vi "GeneralDataRequest new.vi"(6 "Enable":bool, 7 "Ring":u16(ring) items=["PID filter"=3, "Normalized"=2, "Averaged"=1, "RAW"=0], 8 "error in (no error)":errorcluster, 10 "Cluster":T1, 11 "VISA Refnum in":refnum<visa-resource-name>) -> (0 "error out":errorcluster, 3 "Holding Registers":dbl[](array[numeric]))   [LabVIEW 2020]
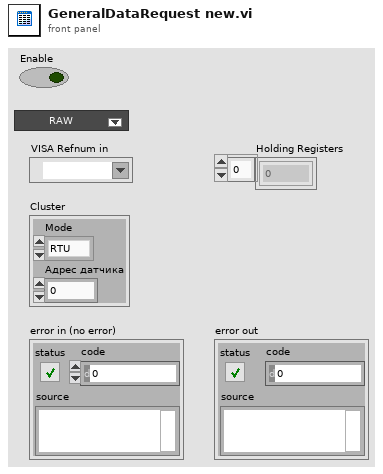
[diagram p1: front panel]
types:
  T1 = cluster{"Mode":enum16{"RTU", "ASCII"}, "Адрес датчика":u16}
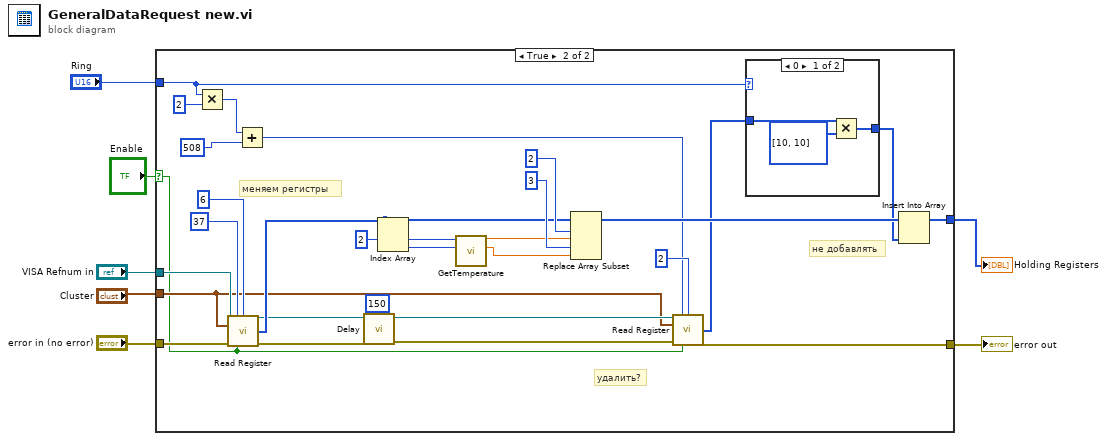
[diagram p0: block diagram]
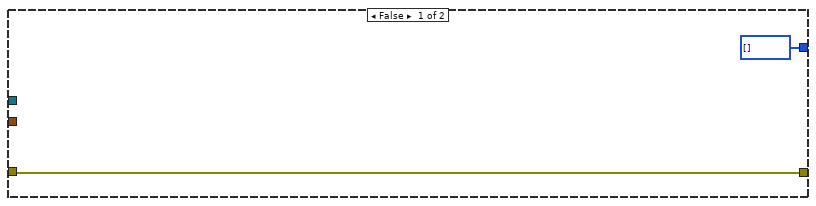
[diagram p2: hidden frame]
diagram:
  n1 = case shown="True" "Enable" {
    selector: "Enable" -> [_ w10]
    tunnel: "error in (no error)" -> [w9 w37]
    tunnel: "VISA Refnum in" -> [_ w36]
    tunnel: "Cluster" -> [_ w21]
    tunnel: [i32[] [] ("Holding Registers") w19] -> w4
    tunnel: [w9 w18] -> w3
    tunnel: "Ring" -> [_ w13]
    frame False {
    }
    frame True {
      # "не добавлять"
      # "удалить?"
      # "меняем регистры"
      n2 = Multiply(x=w13, y=u16 2) -> (x*y=w14:u16)
      n3 = call "Read Register.vi"("Refnum in"=w36, "startReg"=u16 37 ("Holding Register"), "Quantity"=u16 6 ("Holding Register"), "Mode"=w21, "error in (no error)"=w37, "Enable"=w10) -> ("Refnum Out"=w25:refnum<visa-resource-name>, "Holding Registers"=w28:i32[], "error out"=w24:errorcluster)  [unwired: 5 in, 2 out]
      n4 = Add(x=w14, y=u16 508 ("Holding Register")) -> (x+y=w16:u16)
      n5 = call "Delay.vi"("milliseconds to wait"=u32 150, "error in (no error)"=w24, "VISA Refnum  In"=w25) -> ("error out"=w23:errorcluster, "VISA Refnum out"=w22:refnum<visa-resource-name>)  [unwired: 7 in]
      n6 = Index Array(array=w28, index #1=2 ("index")) -> (element #1=w34:i32, element #2=w33:i32)  [unwired: 1 in]
      n7 = call "GetTemperature.vi"("HeaterIn"=w33, "PyroIn"=w34) -> ("HeaterTemp"=w29:dbl, "PyroTemp"=w30:dbl)  [unwired: 8 in]
      n8 = Replace Array Subset(array=w28, new element #1=w30, index #1=2 ("index"), new element #2=w29, index #2=3 ("index")) -> (w20:i32[])
      n9 = call "Read Register.vi"("Refnum in"=w22, "startReg"=w16, "Quantity"=u16 2 ("Holding Register"), "Mode"=w21, "error in (no error)"=w23, "Enable"=w10) -> ("Holding Registers"=w12:i32[], "error out"=w18:errorcluster)  [unwired: 5 in, 3 out]
      n10 = case shown="0" w13 {
        tunnel: w12 -> [w42 w43]
        tunnel: [w40 w43] -> w11
        frame 0 {
          n11 = Multiply(x=w42, y=i32[] [10, 10]) -> (x*y=w40:i32[])
        }
        frame 1, Default {
        }
      }
      n12 = Insert Into Array(array=w20, new element=w11) -> (w19:i32[])  [unwired: 1 in]
    }
  }
  "error out" <- w3
  "Holding Registers" <- w4
